vi "Create_Trajectory_Prepare_Graph.vi"(10 "TRAJECTORY":T1 {"States"."POSE"."ROTATION"."SIN" format="%13.4f"; "States"."POSE"."ROTATION"."COS" format="%13.4f"; "States"."POSE"."ROTATION"."VALUE" format="%13.4f"; "States"."POSE"."TRANSLATION"."Y" format="%14.3f"; "States"."POSE"."TRANSLATION"."X" format="%14.3f"; "TotalTImeSecs" format="%20.3f"}) -> (3 "Array":cluster{dbl[], dbl[]}[](array[cluster]))   [LabVIEW 2019]
uses:
  <vilib>/Rock Robotics/WPI/ThirdParty/JAS_Junk/TrajLib/TypeDef/TRAJECTORY.ctl
  <vilib>/Rock Robotics/WPI/ThirdParty/JAS_Junk/TrajLib/TypeDef/TRAJ_STATE.ctl
  <vilib>/Rock Robotics/WPI/ThirdParty/JAS_Junk/TrajLib/TypeDef/POSE2D.ctl
  <vilib>/Rock Robotics/WPI/ThirdParty/JAS_Junk/TrajLib/TypeDef/TRANSLATION2D.ctl
  <vilib>/Rock Robotics/WPI/ThirdParty/JAS_Junk/TrajLib/TypeDef/ROTATION2D.ctl
  <vilib>/Rock Robotics/WPI/ThirdParty/JAS_Junk/TrajLib/Trajectory_Library.lvlib
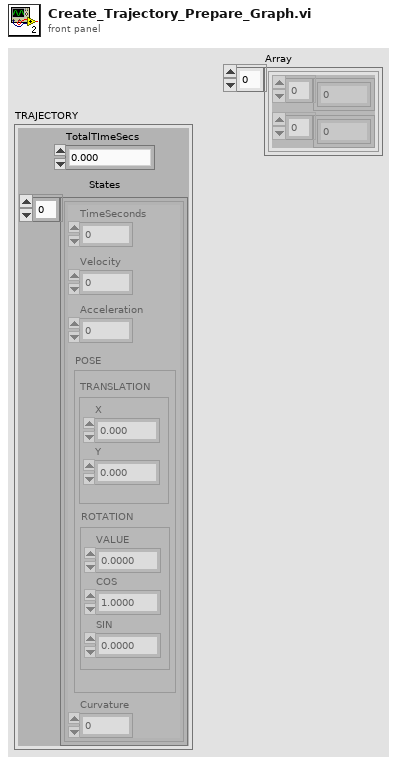
[diagram p1: front panel]
types:
  T1 = typedef "Trajectory_Library.lvlib/TRAJECTORY.ctl" = cluster{"TotalTImeSecs":dbl, "States":T2[]}
  T2 = typedef "Trajectory_Library.lvlib/TRAJ_STATE.ctl" = cluster{"TimeSeconds":dbl, "Velocity":dbl, "Acceleration":dbl, "POSE":T3, "Curvature":dbl}
  T3 = typedef "Trajectory_Library.lvlib/POSE2D.ctl" = cluster{"TRANSLATION":T4, "ROTATION":T5}
  T4 = typedef "Trajectory_Library.lvlib/TRANSLATION2D.ctl" = cluster{"X":dbl, "Y":dbl}
  T5 = typedef "Trajectory_Library.lvlib/ROTATION2D.ctl" = cluster{"VALUE":dbl, "COS":dbl, "SIN":dbl}
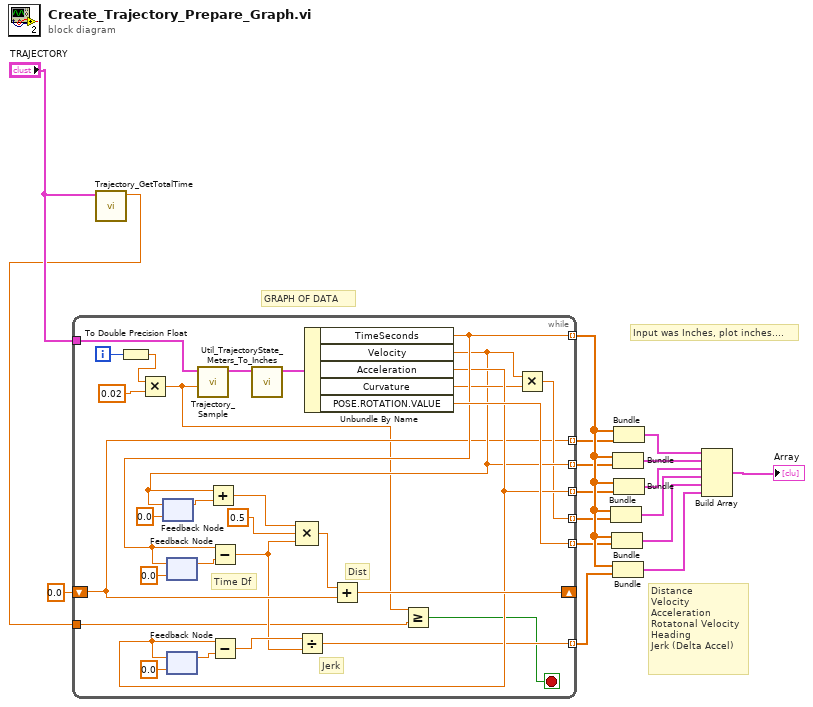
[diagram p0: block diagram]
diagram:
  # "Input was Inches, plot inches...."
  # "Distance\nVelocity\nAcceleration\nRotatonal Velocity\nHeading\nJerk (Delta Accel)"
  # "GRAPH OF DATA"
  n1 = call <vilib>:"Trajectory_GetTotalTime.vi"("TRAJECTORY"="TRAJECTORY") -> ("TotalTime_Sec"=w1:dbl)  [unwired: 10 in]
  n2 = while {
    tunnel: [w39] -> w16 mode=indexing
    tunnel: [w30] -> w6 mode=indexing
    tunnel: [w32] -> w7 mode=indexing
    tunnel: [w36] -> w8 mode=indexing
    tunnel: [w31] -> w9 mode=indexing
    tunnel: [w46] -> w10 mode=indexing
    shift-right: [w40] -> _
    shift-left: 0.0 -> [w30]
    tunnel: [w34] -> w17 mode=indexing
    tunnel: w1 -> [w26]
    tunnel: "TRAJECTORY" -> [w18]
    i -> [w24]
    stop <- w25 stop-if-true
    # "Time Df"
    # "Jerk"
    # "Dist"
    n3 = To Double Precision Float(number=w24) -> (double precision float=w23:dbl)
    n4 = Multiply(x=w23, y=0.02) -> (x*y=w21:dbl)
    n5 = feedback #1(0.0 ("TimeSeconds")) -> (w42:dbl)
    n6 = feedback #2(0.0 ("TimeSeconds")) -> (w44:dbl)
    n7 = feedback #3(0.0 ("TimeSeconds")) -> (w37:dbl)
    n8 = call <vilib>:"Trajectory_Sample.vi"("Time"=w21, "InputTRAJECTORY"=w18) -> ("OutputTRAJ_STATE"=w19:T2)  [unwired: 9 in]
    n9 = call <vilib>:"Util_TrajectoryState_Meters_To_Inches.vi"("absTRAJECTORY"=w19) -> ("outputRelativeTRAJECTORY"=w20:T2)  [unwired: 10 in]
    n10 = Unbundle By Name(w20) -> ("TimeSeconds"=w39:dbl, "Velocity"=w32:dbl, "Acceleration"=w36:dbl, "Curvature"=w33:dbl, "POSE.ROTATION.VALUE"=w46:dbl)
    n11 = feedback-in #1(w32) -> ()
    n12 = feedback-in #2(w39) -> ()
    n13 = feedback-in #3(w36) -> ()
    n14 = Add(x=w32, y=w42) -> (x+y=w41:dbl)
    n15 = Subtract(x=w39, y=w44) -> (x-y=w27:dbl)
    n16 = Subtract(x=w36, y=w37) -> (x-y=w35:dbl)
    n17 = Compound Arithmetic op=MULTIPLY(w41, 0.5 ("value"), w27) -> (w29:dbl)
    n18 = Divide(x=w35, y=w27) -> (x/y=w34:dbl)
    n19 = Add(x=w29, y=w30) -> (x+y=w40:dbl)
    n20 = Greater Or Equal?(x=w21, y=w26) -> (x >= y?=w25:bool)
    n21 = Multiply(x=w32, y=w33) -> (x*y=w31:dbl)
  }
  n22 = Bundle(w16, w9) -> (w11:cluster{dbl[], dbl[]})  [unwired: 1 in]
  n23 = Bundle(w16, w10) -> (w12:cluster{dbl[], dbl[]})  [unwired: 1 in]
  n24 = Bundle(w16, w7) -> (w4:cluster{dbl[], dbl[]})  [unwired: 1 in]
  n25 = Bundle(w16, w17) -> (w15:cluster{dbl[], dbl[]})  [unwired: 1 in]
  n26 = Bundle(w16, w6) -> (w3:cluster{dbl[], dbl[]})  [unwired: 1 in]
  n27 = Bundle(w16, w8) -> (w5:cluster{dbl[], dbl[]})  [unwired: 1 in]
  n28 = Build Array(w3, w4, w5, w11, w12, w15) -> (→"Array":cluster{dbl[], dbl[]}[])
